vi "LogExpSD.vi"(1 "error in (no error)":errorcluster, 2 "II channel seq":T1, 3 "I channel seq":T1, 4 "File":path) -> (0 "error out":errorcluster)   [LabVIEW 2015]
uses:
  controls/data-cluster.ctl
  globalVarSD.vi
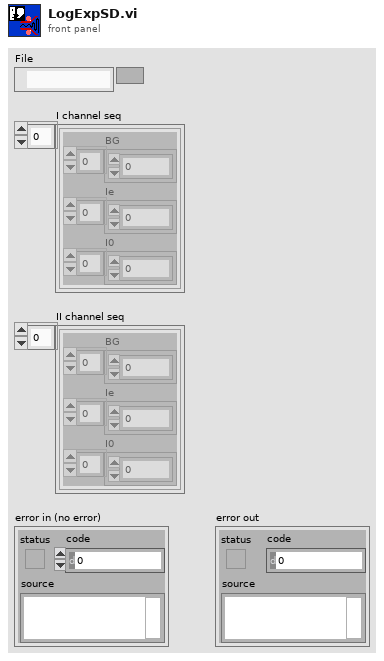
[diagram p1: front panel]
types:
  T1 = typedef "data-cluster.ctl" = cluster{"BG":i32[], "Ie":i32[], "I0":i32[]}[]
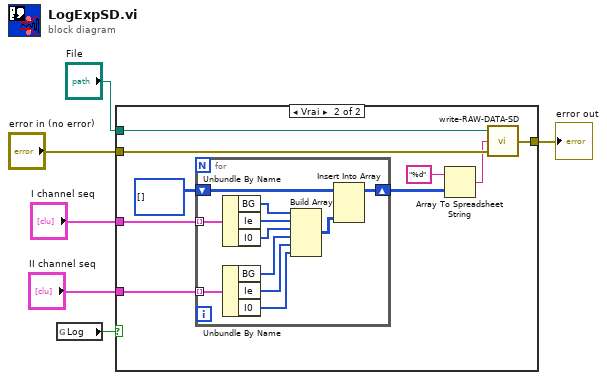
[diagram p0: block diagram]
diagram:
  n1 = global read "globalVarSD.vi" "Log"() -> (w3:bool)
  n2 = case shown="Vrai" w3 {
    tunnel: "I channel seq" -> [_ w10]
    tunnel: "II channel seq" -> [_ w9]
    tunnel: "File" -> [_ w16]
    tunnel: [w7 w15] -> w5
    tunnel: "error in (no error)" -> [w7 w14]
    frame False {
    }
    frame True {
      n3 = for {
        shift-right: [w20] -> w13
        shift-left: i32[][] [] -> [w21]
        tunnel: w10 -> [w19] mode=indexing
        tunnel: w9 -> [w18] mode=indexing
        n4 = Unbundle By Name(w19) -> ("BG"=w27:i32[], "Ie"=w26:i32[], "I0"=w25:i32[])
        n5 = Unbundle By Name(w18) -> ("BG"=w24:i32[], "Ie"=w23:i32[], "I0"=w22:i32[])
        n6 = Build Array(w27, w26, w25, w24, w23, w22) -> (w17:i32[][])
        n7 = Insert Into Array(array=w21, new element=w17) -> (w20:i32[][])  [unwired: 2 in]
      }
      n8 = Array To Spreadsheet String(array=w13, 3:"%d" ("format string")) -> (spreadsheet string=w8:string)  [unwired: 1 in]
      n9 = call "write-RAW-DATA-SD.vi"("error in (no error)"=w14, "Text"=w8, "File"=w16) -> ("error out"=w15:errorcluster)
    }
  }
  "error out" <- w5
